vi "oa_Tachless Popup Position Modification.vi"(9 "Pop Area":T1, 10 "mouse position":cluster{"left":i32, "top":i32}, 11 "Popup Menu":refnum<vi>) -> (2 "position":cluster{i32, i32}, 3 "dup Popup Menu":refnum<vi>)   [LabVIEW 2017, in "SoundVib_Tachless.lvlib"]
uses:
  <vilib>/addons/Sound and Vibration/Order Analysis/Tachless/SoundVib_Tachless.lvlib
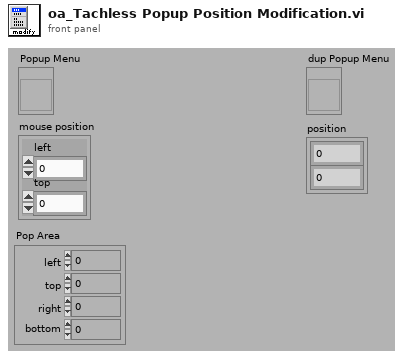
[diagram p1: front panel]
types:
  T1 = cluster{"left":i16, "top":i16, "right":i16, "bottom":i16}
  T2 = typedef "LVBoundsTypeDef.ctl" = cluster{"Width":u32, "Height":u32}
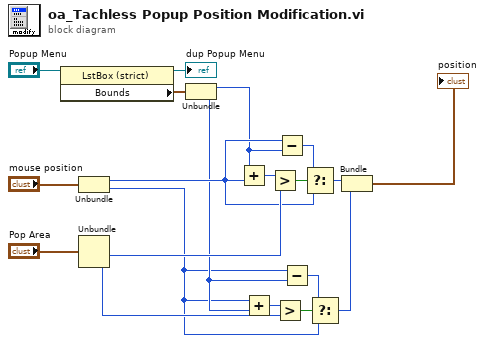
[diagram p0: block diagram]
diagram:
  n1 = property class="LstBox (strict)"(reference="Popup Menu") -> (reference out=→"dup Popup Menu":refnum<vi>, "Bounds"=w17:T2)  [unwired: 1 in, 1 out]
  n2 = Unbundle("mouse position") -> ("left"=w13:i32, "top"=w1:i32)
  n3 = Unbundle("Pop Area") -> ("right"=w15:i16, "bottom"=w4:i16)  [unwired: 2 out]
  n4 = Unbundle(w17) -> ("Width"=w12:u32, "Height"=w2:u32)
  n5 = Add(x=w12, y=w13) -> (x+y=w16:u32)
  n6 = Add(x=w1, y=w2) -> (x+y=w8:u32)
  n7 = Greater?(x=w16, y=w15) -> (0:w14:bool)
  n8 = Greater?(x=w8, y=w4) -> (0:w9:bool)
  n9 = Subtract(x=w13, y=w12) -> (x-y=w11:u32)
  n10 = Subtract(x=w1, y=w2) -> (x-y=w10:u32)
  n11 = Select(t=w11, s=w14, f=w13) -> (s? t:f=w7:u32)
  n12 = Select(t=w10, s=w9, f=w1) -> (s? t:f=w6:u32)
  n13 = Bundle("left"=w7, "top"=w6) -> (→"position":cluster{"left":u32, "top":u32})  [unwired: 1 in]
